vi "Get Scale Error.vi"(8 "error in (no error)":errorcluster, 11 "VISA resource name":refnum<visa-resource-name>) -> (0 "error out":errorcluster, 1 "Scale Error Units":i32, 2 "Scale Error":dbl format="%^.3e", 3 "VISA resource name out":refnum<visa-resource-name>)   [LabVIEW 2013, in "Fluke 5XXX Series Multicalibrators.lvlib"]
doc: "This VI returns the value of the scale error if scaling is on; otherwise, this command returns 0.0.\n\nNote:\n\nThis VI is available only for instrument models 5700A and 5720A."
uses:
  Fluke 5XXX Series Multicalibrators.lvlib
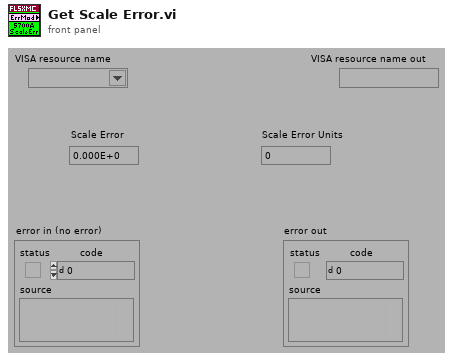
[diagram p1: front panel]
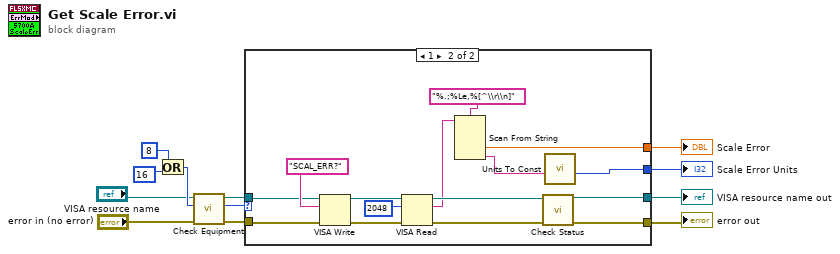
[diagram p0: block diagram]
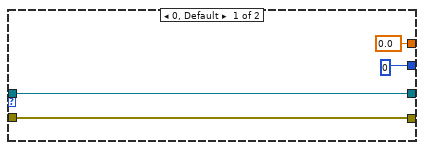
[diagram p2: hidden frame]
diagram:
  n1 = Or(x=8 ("Numeric"), y=16 ("Numeric")) -> (x .or. y?=w7:i32)
  n2 = call "Check Equipment.vi"("error in (no error)"="error in (no error)", "Bit Mask"=w7, "VISA resource name"="VISA resource name") -> ("error out"=w12:errorcluster, "Present?"=w11:u32, "VISA resource name out"=w10:refnum<visa-resource-name>)  [unwired: 6 in]
  n3 = case shown="1" w11 {
    tunnel: [w16 w25] -> w3
    tunnel: [w15 w22] -> w4
    tunnel: w12 -> [w16 w27]
    tunnel: w10 -> [w15 w26]
    tunnel: [0.0 w19] -> w1
    tunnel: [u16 0 w18] -> w2
    frame 0, Default {
    }
    frame 1 {
      n4 = VISA Write(VISA resource name=w26, write buffer="SCAL_ERR?", error in (no error)=w27) -> (VISA resource name out=w30:refnum<visa-resource-name>, error out=w29:errorcluster)  [unwired: 1 out]
      n5 = VISA Read(VISA resource name=w30, byte count=u32 2048 ("byte count (0)"), error in (no error)=w29) -> (VISA resource name out=w23:refnum<visa-resource-name>, read buffer=w20:string, error out=w24:errorcluster)  [unwired: 1 out]
      n6 = Scan From String(format string="%.;%Le,%[^\\r\\n]", input string=w20) -> (output 1=w19:dbl, output 2=w17:string)  [unwired: 4 in, 3 out]
      n7 = call "Check Status.vi"("VISA resource name"=w23, "error in (no error)"=w24) -> ("VISA resource name out"=w22:refnum<visa-resource-name>, "error out"=w25:errorcluster)  [unwired: 12 in]
      n8 = call "Units To Const.vi"("Units"=w17) -> ("Const"=w18:i32)  [unwired: 10 in]
    }
  }
  "Scale Error" <- w1
  "Scale Error Units" <- w2
  "VISA resource name out" <- w4
  "error out" <- w3
